vi "LoadPicture.vi"(8 "error in (no error)":errorcluster, 11 "path to PNG file":path=path "/home/lvuser/natinst/bin/data/Aesomatica_16x16.png") -> (0 "error out":errorcluster, 3 "Image Pixels (U64)":T1[][](array[typedef]))   [LabVIEW 2019, in "RT_Game.lvlib" / "Game.lvclass"]
uses:
  Game.lvclass
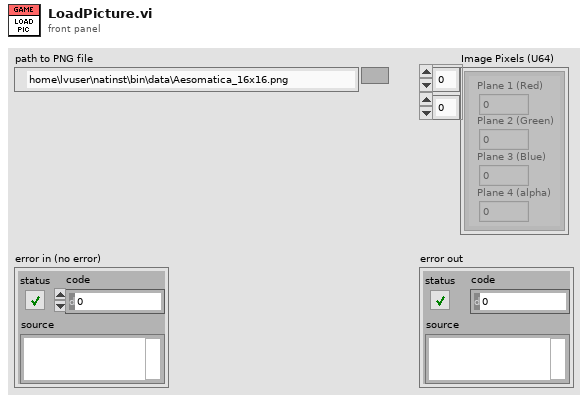
[diagram p1: front panel]
types:
  T1 = typedef "Color (U64)" = cluster{"Plane 3 (Blue)":u16, "Plane 2 (Green)":u16, "Plane 1 (Red)":u16, "Plane 4 (alpha)":u16}
  T2 = typedef "Image Type" = u32
  T3 = typedef "IMAQ Image.ctl" = refnum<image>
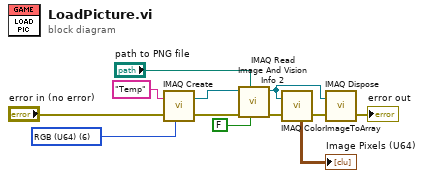
[diagram p0: block diagram]
diagram:
  w11 = T2 6 items=["Grayscale (U8)", "Grayscale (I16)", "Grayscale (SGL)", "Complex (CSG)", "RGB (U32)", "HSL (U32)", "RGB (U64)", "Grayscale (U16)"] ("Image Type")
  n1 = call "IMAQ Create"("Image Name"="Temp", "Image Type"=w11, "error in (no error)"="error in (no error)") -> ("New Image"=w9:T3, "error out"=w8:errorcluster)  [unwired: 2 in]
  n2 = call "IMAQ Read Image And Vision Info 2"("Use File Path Image Type"=FALSE, "File Path"="path to PNG file", "error in (no error)"=w8, "Image"=w9) -> ("error out"=w7:errorcluster, "Image Out"=w5:T3)  [unwired: 5 in, 1 out]
  n3 = call "IMAQ ColorImageToArray"("Image"=w5, "error in (no error)"=w7) -> ("error out"=w6:errorcluster, "Image Pixels (U64)"=→"Image Pixels (U64)":T1[][])  [unwired: 2 in, 1 out]
  n4 = call "IMAQ Dispose"("Image"=w5, "error in (no error)"=w6) -> ("error out"=→"error out":errorcluster)  [unwired: 4 in]
